vi "Stream Data I64x2.vi"(0 "i in":fxp<+/-,64,1>, 1 "clear overflow":bool, 5 "q in":fxp<+/-,64,1>, 7 "config":T3, 9 "input valid":bool) -> (6 "status":T2, 10 "overflow?":bool)   [LabVIEW 2018, in "Lock-In Amplifier Example FPGA.lvlib"]
uses:
  Lock-In Amplifier Example FPGA.lvlib
  <instrlib>/_niInstr/Streaming/v1/Common/Stream State.ctl
  <vilib>/rvi/interface/RandomDataEmulation/niFpgaRandomDataHandleErrors.vi
  <vilib>/rvi/DataTransferAndStorage/Container/XNode/niFpgaContainer.xnode
  <vilib>/rvi/interface/RandomDataEmulation/nirviRandomDataFpgaReadWriteTemplate.vi
  <instrlib>/_niInstr/Streaming/v1/FPGA/niInstr Streaming v1 FPGA.lvlib
  <instrlib>/_niInstr/Basic Elements/v1/FPGA/niInstr Basic Elements v1 FPGA.lvlib
  <instrlib>/_niInstr/Streaming/v1/Common/niInstr Streaming v1 Common.lvlib
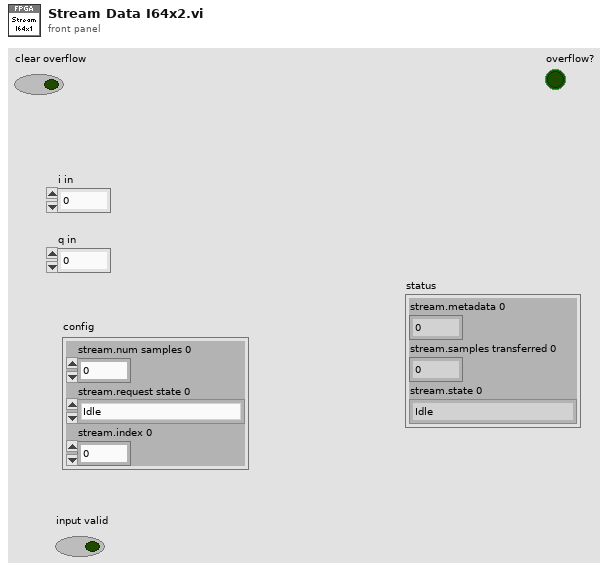
[diagram p1: front panel]
types:
  T1 = typedef "niInstr Streaming v1 Common.lvlib/Stream State.ctl" = enum8{"Idle", "Finite Transfer", "Continuous", "Done", "Error", "Not Ready", "Cancel"}
  T2 = cluster{"stream.metadata 0":u64, "stream.samples transferred 0":u64, "stream.state 0":T1}
  T3 = cluster{"stream.num samples 0":u64, "stream.request state 0":T1, "stream.index 0":i16}
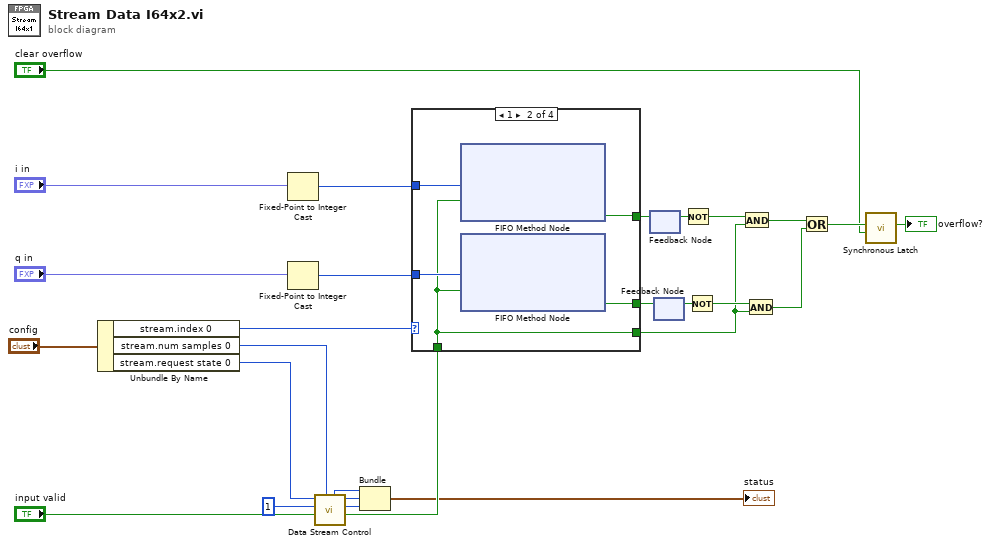
[diagram p0: block diagram]
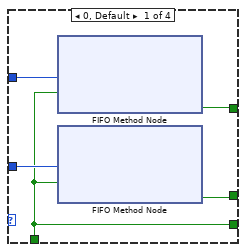
[diagram p2: hidden frame]
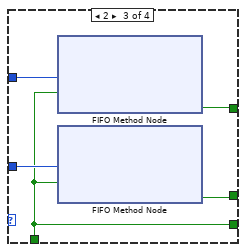
[diagram p3: hidden frame]
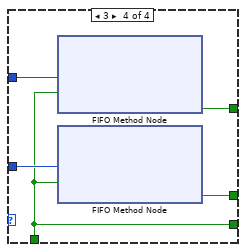
[diagram p4: hidden frame]
diagram:
  n1 = Unbundle By Name("config") -> ("stream.index 0"=w13:i16, "stream.num samples 0"=w19:u64, "stream.request state 0"=w18:T1)
  n2 = Fixed-Point to Integer Cast(1:"i in") -> (0:w24:i64)
  n3 = Fixed-Point to Integer Cast(1:"q in") -> (0:w22:i64)
  n4 = call <instrlib>:"Data Stream Control.vi"("stream.num samples 0"=w19, "data valid"="input valid", "element count"=u16 1, "stream.request state 0"=w18) -> ("send data"=w21:bool, "stream.state 0"=w15:T1, "stream.samples transferred 0"=w16:u64, "stream.metadata 0"=w17:u64)  [unwired: 3 in, 1 out]
  n5 = Bundle("stream.metadata 0"=w17, "stream.samples transferred 0"=w16, "stream.state 0"=w15) -> (→"status":T2)  [unwired: 1 in]
  n6 = case shown="1" w13 {
    tunnel: w24 -> [w32 w37 w42 w47]
    tunnel: w22 -> [w31 w36 w41 w46]
    tunnel: w21 -> [w29 w34 w39 w44]
    tunnel: [w30 w35 w40 w45] -> w10
    tunnel: [w29 w34 w39 w44] -> w6
    tunnel: [w28 w33 w38 w43] -> w9
    frame 0, Default {
      n7 = xnode ("FIFO Method Node")("Element"=w32, "Input Valid"=w29) -> ("Ready for Input"=w28:bool)  [unwired: 1 in, 1 out]
      n8 = xnode ("FIFO Method Node")("Element"=w31, "Input Valid"=w29) -> ("Ready for Input"=w30:bool)  [unwired: 1 in, 1 out]
    }
    frame 1 {
      n9 = xnode ("FIFO Method Node")("Element"=w37, "Input Valid"=w34) -> ("Ready for Input"=w33:bool)  [unwired: 1 in, 1 out]
      n10 = xnode ("FIFO Method Node")("Element"=w36, "Input Valid"=w34) -> ("Ready for Input"=w35:bool)  [unwired: 1 in, 1 out]
    }
    frame 2 {
      n11 = xnode ("FIFO Method Node")("Element"=w42, "Input Valid"=w39) -> ("Ready for Input"=w38:bool)  [unwired: 1 in, 1 out]
      n12 = xnode ("FIFO Method Node")("Element"=w41, "Input Valid"=w39) -> ("Ready for Input"=w40:bool)  [unwired: 1 in, 1 out]
    }
    frame 3 {
      n13 = xnode ("FIFO Method Node")("Element"=w47, "Input Valid"=w44) -> ("Ready for Input"=w43:bool)  [unwired: 1 in, 1 out]
      n14 = xnode ("FIFO Method Node")("Element"=w46, "Input Valid"=w44) -> ("Ready for Input"=w45:bool)  [unwired: 1 in, 1 out]
    }
  }
  n15 = feedback #1() -> (w8:bool)  [unwired: 1 in]
  n16 = feedback-in #1(w9) -> ()
  n17 = feedback #2() -> (w12:bool)  [unwired: 1 in]
  n18 = feedback-in #2(w10) -> ()
  n19 = Not(x=w8) -> (.not. x?=w7:bool)
  n20 = Not(x=w12) -> (.not. x?=w11:bool)
  n21 = And(x=w7, y=w6) -> (x .and. y?=w5:bool)
  n22 = And(x=w11, y=w6) -> (x .and. y?=w4:bool)
  n23 = Or(x=w5, y=w4) -> (x .or. y?=w3:bool)
  n24 = call <instrlib>:"Synchronous Latch.vi"("clear"="clear overflow", "set"=w3) -> ("out"=→"overflow?":bool)  [unwired: 9 in]
